vi "shag_start — 3.vi"() -> ()   [LabVIEW 2016]
uses:
  <vilib>/Instr/_visa.llb/VISA Configure Serial Port (Instr).vi
panel:
  in  "Блокировать зеркало №1":bool
  out "положение в мин 1":i32
  in  "stop":bool
  in  "all":T1(tab)
  out "положение шд":i32(knob) scale=-10.0..190.0
  out "текущее положение":string
  out "положение в минутах 1":string
  in  "Минуты":i32 min=-600 max=11400
  in  "Stop двигатель":bool
  in  "Вращение по градусам +":bool
  in  "Вращение по градусам -":bool
  in  "Вернуться в нулевое положение":bool
  in  "Задать текущее положение нулевым":bool
  in  "Установка минут":bool
  in  "Выберете COM порт":refnum<visa-resource-name>="COM1"
  in  "Скорость обмена данными":u32(ring)=19200 items=["9600"=9600, "19200"=19200, "38400"=38400, "57600"=57600]
  in  "Число бит на символ":u16=8 min=5 max=8 step=1
  in  "Контроль чётности":enum16{"None", "Odd", "Even", "Mark", "Space"}(ring)
  in  "Стоповый бит":u16(ring)=10 items=["1.0"=10, "1.5"=15, "2.0"=20]
  in  "Контроль переполнения":u16(ring) items=["None"=0, "XON/XOFF"=1, "RTS/CTS"=2, "DTR/DSR"=4]
  # "1 - адресс 1 двигателя\n2 - адресс 2 двигателя\n$0MV\\01+   - запуск всех двигателей в положительном направлении \n$0MS\\00   - остановка всех двигателей\n$0MJ\\04+\\00\\00\\01   - 1 шаг всех двигателей\n$0SS\\01\\10   - скорость 10 для всех двигателей"
  # "Зеркало №1:"
  # "Положение:"
  # "Ренгеновская трубка №2:"
  # "Положение ренгеновской трубк:"
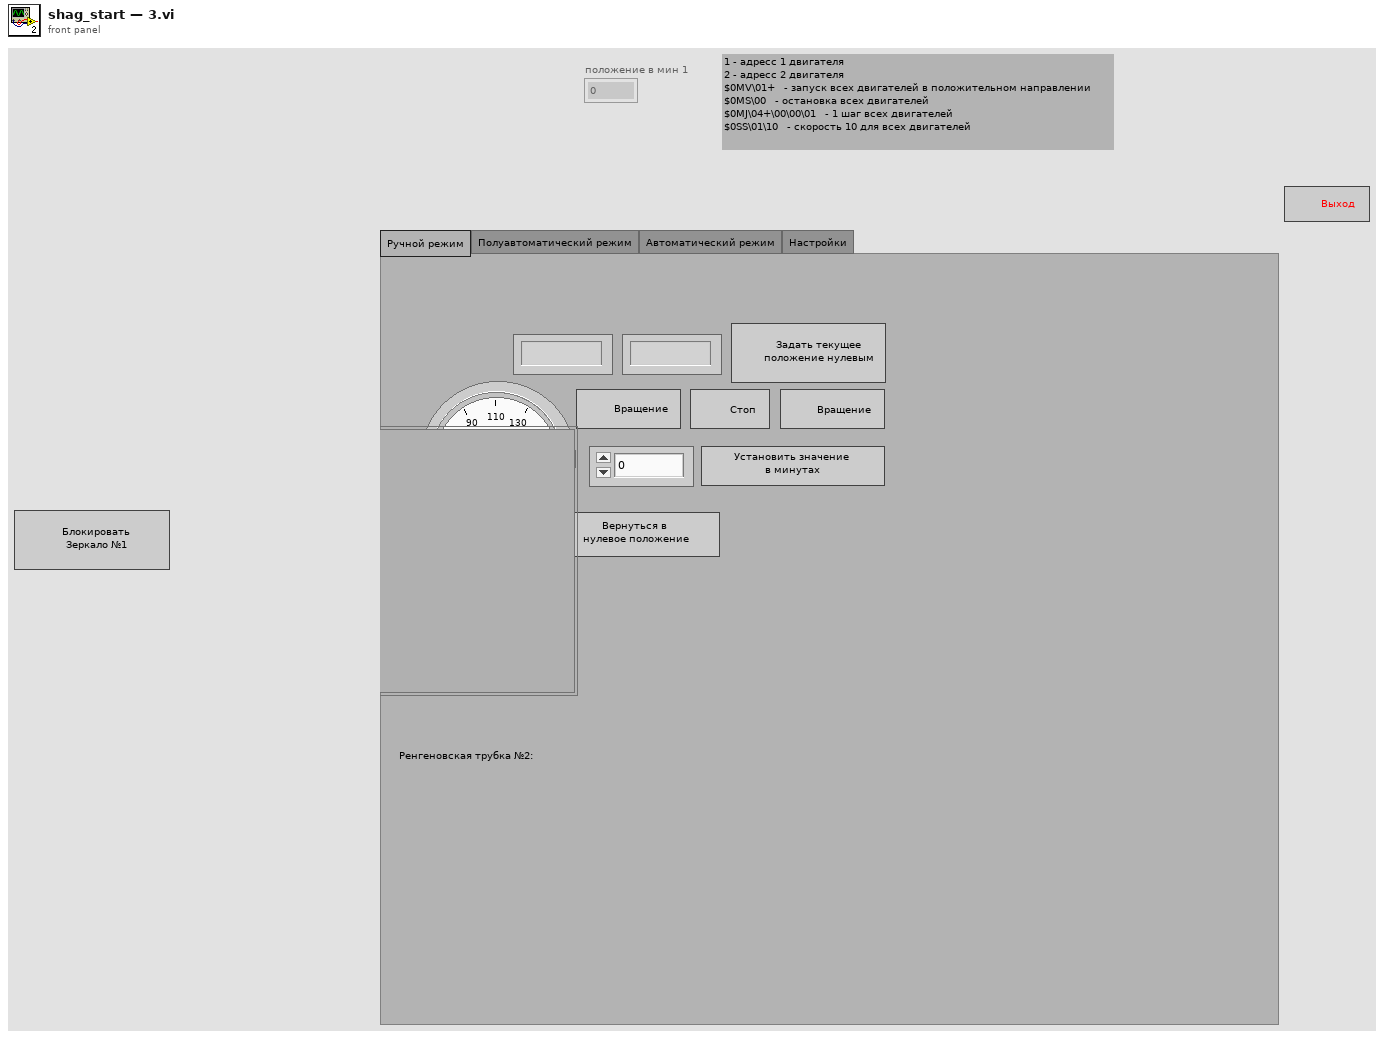
[diagram p1: front panel]
types:
  T1 = enum32{"Ручной режим", "Полуавтоматический режим", "Автоматический режим", "Настройки"}
  T2 = enum8{"Enabled", "Disabled", "Disabled and Grayed Out"}
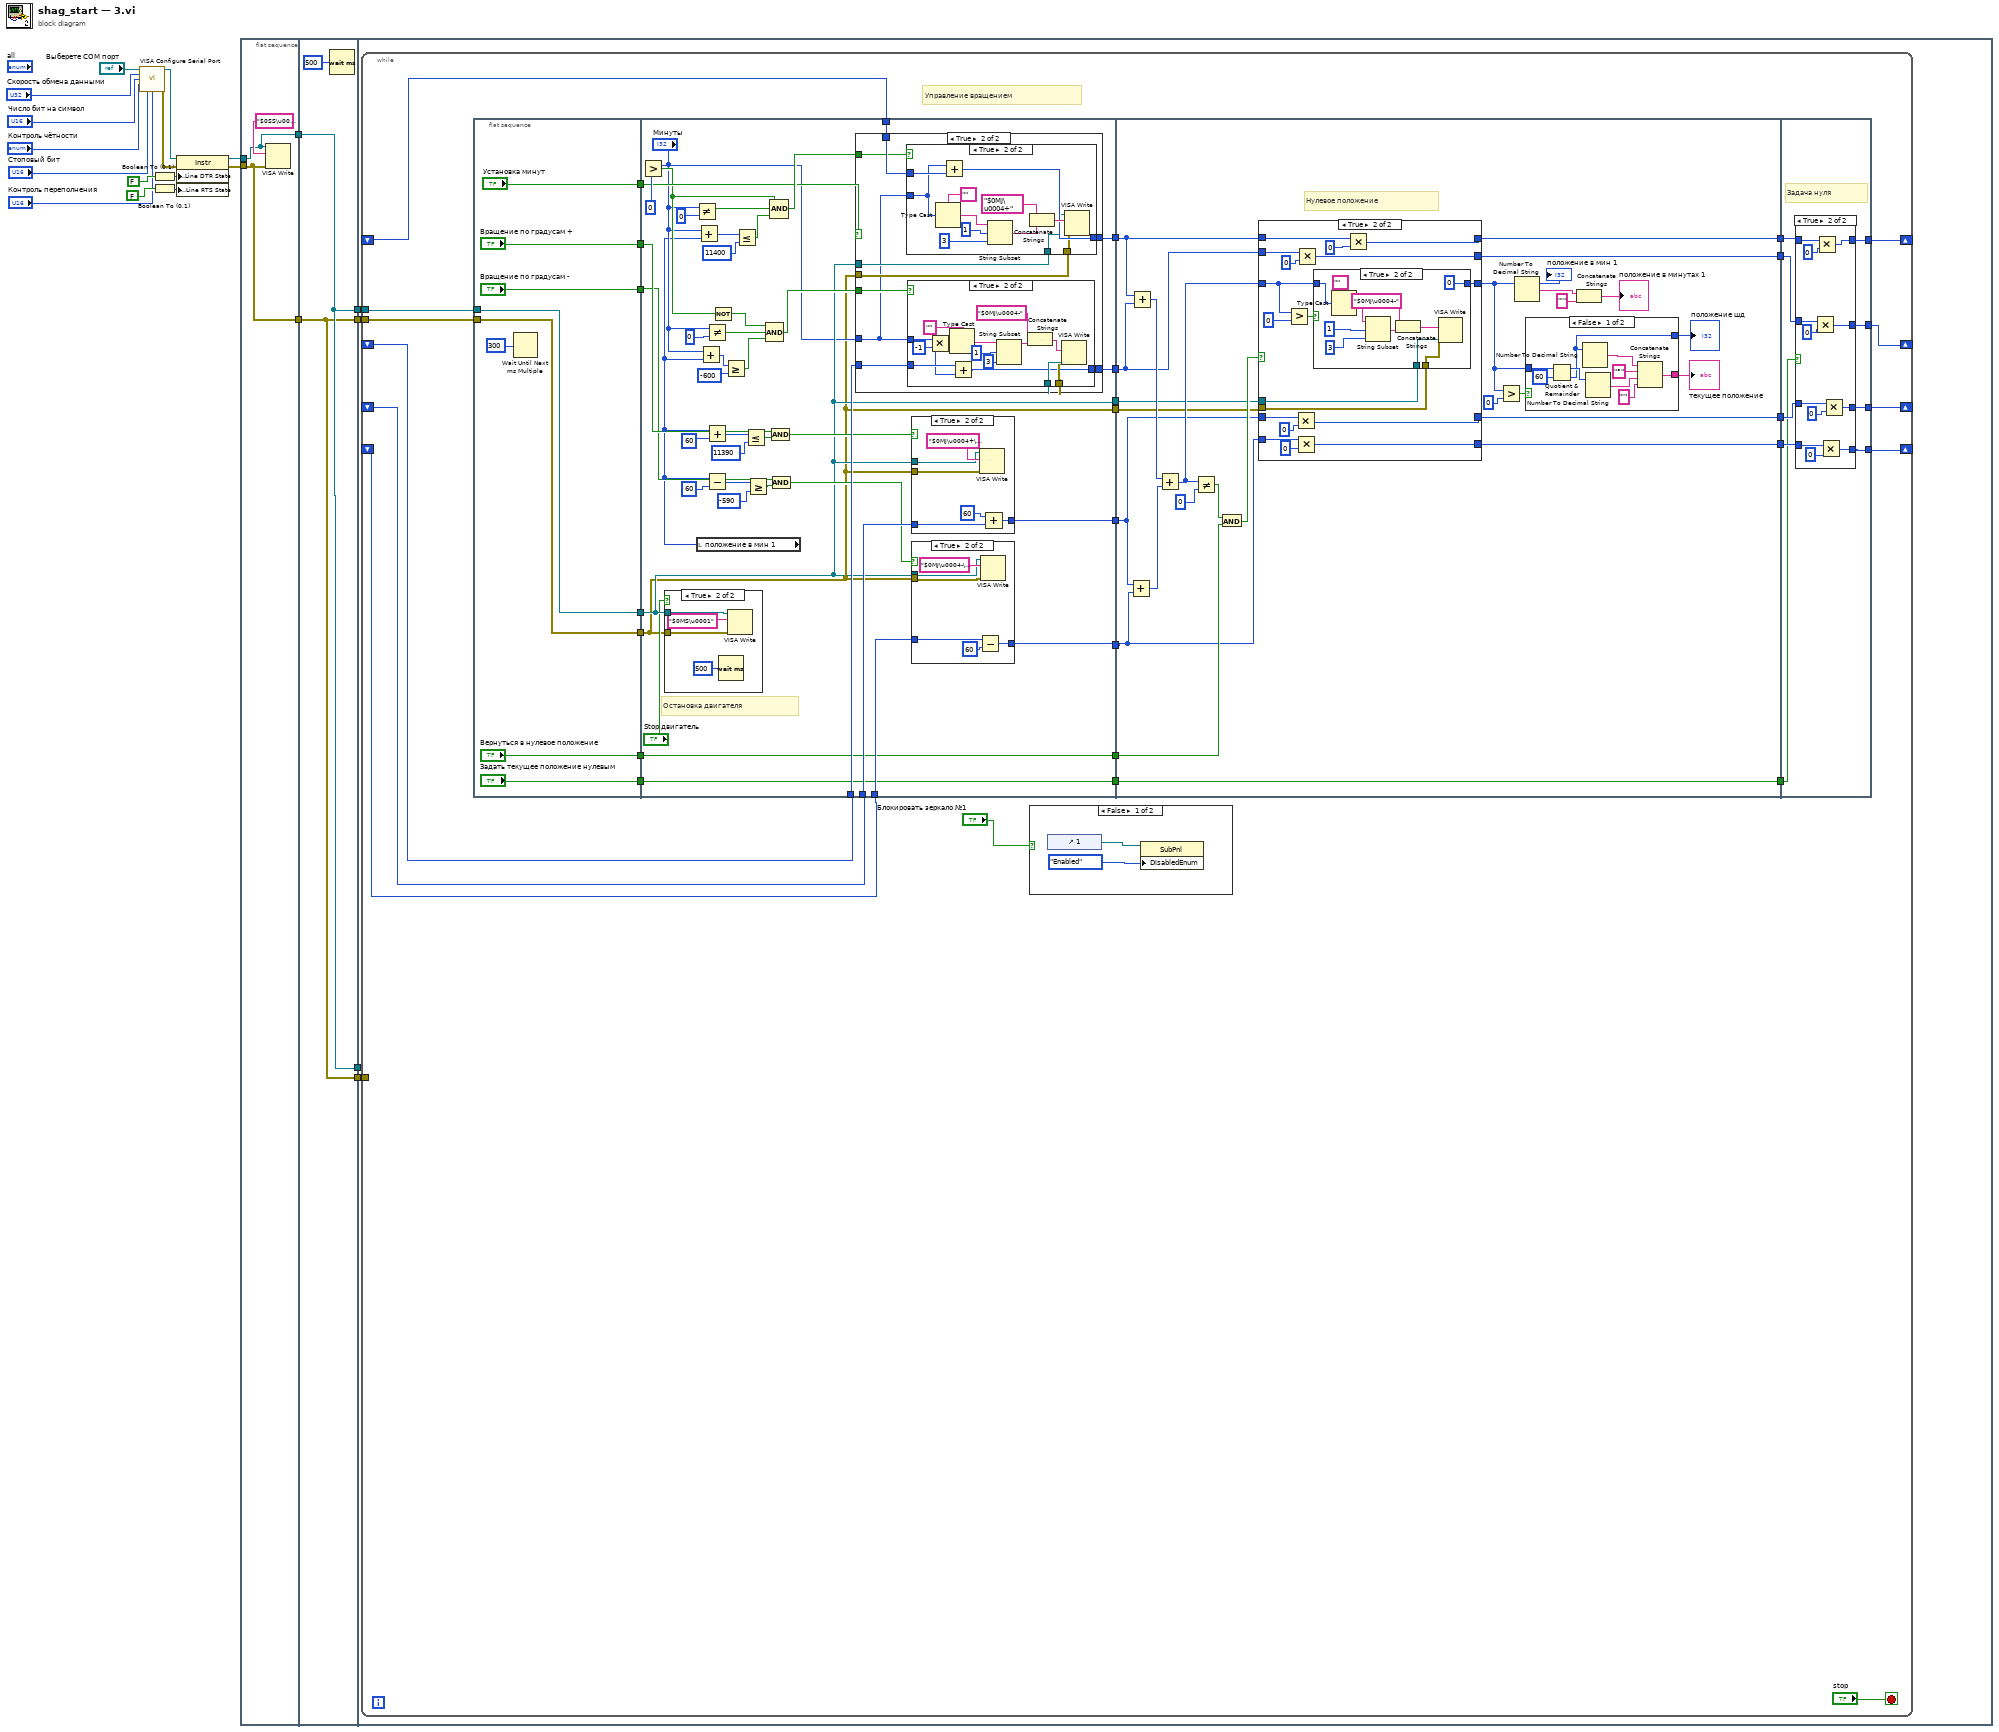
[diagram p0: block diagram]
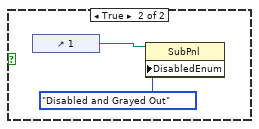
[diagram p2: hidden frame]
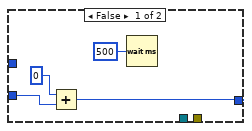
[diagram p4: hidden frame]
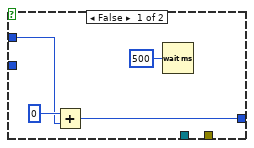
[diagram p5: hidden frame]
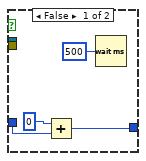
[diagram p7: hidden frame]
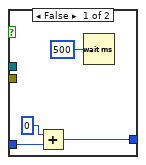
[diagram p8: hidden frame]
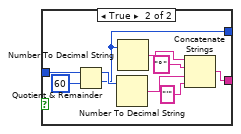
[diagram p9: hidden frame]
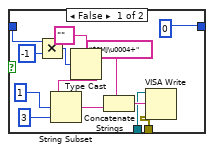
[diagram p11: hidden frame]
diagram:
  n1 = call-poly "VISA Configure Serial Port"("VISA resource name"="Выберете COM порт", "baud rate (9600)"="Скорость обмена данными", "data bits (8)"="Число бит на символ", "parity (0:none)"="Контроль чётности", "stop bits (10: 1 bit)"="Стоповый бит", "flow control (0:none)"="Контроль переполнения") -> ("VISA resource name out"=w18:refnum<visa-resource-name>, "error out"=w17:errorcluster)  [unwired: 8 in]
  n2 = Boolean To (0,1)(Boolean=FALSE ("DTR Write")) -> (0, 1=w19:i16)
  n3 = Boolean To (0,1)(Boolean=FALSE ("DTR Write")) -> (0, 1=w20:i16)
  n4 = property class="Instr"(reference=w18, error in=w17, "Serial Settings:Modem Line Settings:Line DTR State"=w19, "Serial Settings:Modem Line Settings:Line RTS State"=w20) -> (reference out=w16:refnum<visa-resource-name>, error out=w15:errorcluster)
  n5 = flat-sequence {
    tunnel: w16 -> [w22]
    tunnel: w15 -> [w21]
    tunnel: [w22] -> w13
    tunnel: [w21] -> w12
    tunnel: [w25] -> w14
    tunnel: w13 -> [w25]
    tunnel: w12 -> [w24]
    tunnel: [w24] -> w11
    tunnel: [w25] -> w2
    tunnel: [w24] -> w1
    tunnel: w14 -> [w29]
    tunnel: w11 -> [w28]
    tunnel: w2 -> [_]
    tunnel: w1 -> [w27]
    frame #0 {
      n6 = VISA Write(VISA resource name=w22, write buffer="$0SS\u0001\u0010", error in (no error)=w21) -> ()  [unwired: 3 out]
    }
    frame #1 {
      n7 = Wait (ms)(milliseconds to wait=u32 500) -> ()  [unwired: 1 out]
    }
    frame #2 {
      n8 = while {
        tunnel: w29 -> [w36]
        tunnel: w28 -> [w35]
        shift-right: [w31] -> _
        shift-left: _ -> [w40]
        shift-right: [w32] -> _
        shift-left: _ -> [w39]
        shift-right: [w33] -> _
        shift-left: _ -> [w38]
        shift-right: [w34] -> _
        shift-left: _ -> [w37]
        tunnel: w27 -> [_]
        stop <- "stop" stop-if-true
        # "Управление вращением"
        n9 = flat-sequence {
          tunnel: w35 -> [w72]
          tunnel: w36 -> [w73]
          tunnel: [w73] -> w60
          tunnel: [w72] -> w59
          tunnel: ["Вращение по градусам +"] -> w58
          tunnel: ["Вращение по градусам -"] -> w57
          tunnel: ["Вернуться в нулевое положение"] -> w56
          tunnel: ["Задать текущее положение нулевым"] -> w55
          tunnel: ["Установка минут"] -> w54
          tunnel: w60 -> [w93]
          tunnel: w59 -> [w74]
          tunnel: [w116] -> w53
          tunnel: w40 -> [w113]
          tunnel: w39 -> [w115]
          tunnel: [w114] -> w52
          tunnel: w38 -> [w112]
          tunnel: w37 -> [w111]
          tunnel: w58 -> [w97]
          tunnel: w57 -> [w96]
          tunnel: [w110] -> w51
          tunnel: [w109] -> w50
          tunnel: [w94] -> w49
          tunnel: w56 -> [w94]
          tunnel: [w74] -> w48
          tunnel: [w93] -> w47
          tunnel: [w92] -> w46
          tunnel: w55 -> [w92]
          tunnel: w54 -> [w86]
          tunnel: w53 -> [w190]
          tunnel: w52 -> [w191]
          tunnel: [w211] -> w45
          tunnel: [w209] -> w44
          tunnel: w51 -> [w192]
          tunnel: w50 -> [w193]
          tunnel: [w199] -> w43
          tunnel: [w207] -> w42
          tunnel: w49 -> [w203]
          tunnel: w48 -> [w198]
          tunnel: w47 -> [w197]
          tunnel: w46 -> [w195]
          tunnel: [w195] -> w41
          tunnel: [w285] -> w31
          tunnel: [w282] -> w32
          tunnel: w45 -> [w284]
          tunnel: w44 -> [w283]
          tunnel: [w281] -> w33
          tunnel: [w280] -> w34
          tunnel: w43 -> [w279]
          tunnel: w42 -> [w278]
          tunnel: w41 -> [w277]
          frame #0 {
            n10 = Wait Until Next ms Multiple(millisecond multiple=u32 300) -> ()  [unwired: 1 out]
          }
          frame #1 {
            # "Остановка двигателя"
            n11 = Greater?(x="Минуты", y=0) -> (0:w84:bool)
            n12 = case shown="True" "Stop двигатель" {
              tunnel: w93 -> [_ w163]
              tunnel: w74 -> [_ w162]
              frame False {
              }
              frame True {
                n13 = Wait (ms)(milliseconds to wait=u32 500) -> ()  [unwired: 1 out]
                n14 = VISA Write(VISA resource name=w163, write buffer="$0MS\u0001", error in (no error)=w162) -> ()  [unwired: 3 out]
              }
            }
            n15 = Not Equal?(x="Минуты", y=0) -> (x != y?=w83:bool)
            n16 = local read "положение в мин 1"() -> (w79:i32)
            n17 = Add(x="Минуты", y=w79) -> (x+y=w107:i32)
            n18 = Add(x="Минуты", y=w79) -> (x+y=w77:i32)
            n19 = Not Equal?(x="Минуты", y=0) -> (x != y?=w81:bool)
            n20 = Add(x=w79, y=60) -> (x+y=w102:i32)
            n21 = Subtract(x=w79, y=60) -> (x-y=w89:i32)
            n22 = Not(x=w84) -> (.not. x?=w85:bool)
            n23 = Greater Or Equal?(x=w77, y=-600) -> (x >= y?=w78:bool)
            n24 = Less Or Equal?(x=w107, y=11400) -> (x <= y?=w82:bool)
            n25 = Less Or Equal?(x=w102, y=11390) -> (x <= y?=w99:bool)
            n26 = Greater Or Equal?(x=w89, y=-590) -> (x >= y?=w90:bool)
            n27 = Compound Arithmetic op=AND(w85, w81, w78) -> (w103:bool)
            n28 = And(x=w97, y=w99) -> (x .and. y?=w98:bool)
            n29 = And(x=w96, y=w90) -> (x .and. y?=w95:bool)
            n30 = Compound Arithmetic op=AND(w84, w83, w82) -> (w105:bool)
            n31 = case shown="True" w86 {
              tunnel: [w118 w127] -> w116
              tunnel: w115 -> [w117 w126]
              tunnel: [w117 w125] -> w114
              tunnel: w113 -> [w118 w124]
              tunnel: w105 -> [_ w123]
              tunnel: w103 -> [_ w122]
              tunnel: w74 -> [_ w121]
              tunnel: w93 -> [_ w120]
              tunnel: "Минуты" -> [_ w119]
              frame False {
              }
              frame True {
                n32 = case shown="True" w123 {
                  tunnel: [w148 w154] -> w127
                  tunnel: w124 -> [w147 w153]
                  tunnel: w121 -> [_ w152]
                  tunnel: w120 -> [_ w151]
                  tunnel: w119 -> [_ w150]
                  frame False {
                    n33 = Add(x=0, y=w147) -> (x+y=w148:i32)
                    n34 = Wait (ms)(milliseconds to wait=u32 500) -> ()  [unwired: 1 out]
                  }
                  frame True {
                    n35 = Type Cast(type="", x=w150) -> (*(type *) &x=w157:string)
                    n36 = Add(x=w150, y=w153) -> (x+y=w154:i32)
                    n37 = String Subset(string=w157, offset (0)=1, length (rest)=3 ("length (rest)")) -> (substring=w156:string)
                    n38 = Concatenate Strings("$0MJ\u0004+" ("write buffer"), w156) -> (w160:string)
                    n39 = VISA Write(VISA resource name=w151, write buffer=w160, error in (no error)=w152) -> ()  [unwired: 3 out]
                  }
                }
                n40 = case shown="True" w122 {
                  tunnel: [w130 w136] -> w125
                  tunnel: w126 -> [w129 w135]
                  tunnel: w120 -> [_ w138]
                  tunnel: w121 -> [_ w137]
                  tunnel: w119 -> [_ w132]
                  frame False {
                    n41 = Add(x=0, y=w129) -> (x+y=w130:i32)
                    n42 = Wait (ms)(milliseconds to wait=u32 500) -> ()  [unwired: 1 out]
                  }
                  frame True {
                    n43 = Multiply(x=w132, y=-1) -> (x*y=w134:i32)
                    n44 = Type Cast(type="", x=w134) -> (*(type *) &x=w141:string)
                    n45 = Add(x=w135, y=w132) -> (x+y=w136:i32)
                    n46 = String Subset(string=w141, offset (0)=1, length (rest)=3 ("length (rest)")) -> (substring=w140:string)
                    n47 = Concatenate Strings("$0MJ\u0004-" ("write buffer"), w140) -> (w144:string)
                    n48 = VISA Write(VISA resource name=w138, write buffer=w144, error in (no error)=w137) -> ()  [unwired: 3 out]
                  }
                }
              }
            }
            n49 = case shown="True" w98 {
              tunnel: [w178 w185] -> w110
              tunnel: w112 -> [w177 w180]
              tunnel: w93 -> [_ w181]
              tunnel: w74 -> [_ w182]
              frame False {
                n50 = Add(x=0, y=w177) -> (x+y=w178:i32)
                n51 = Wait (ms)(milliseconds to wait=u32 500) -> ()  [unwired: 1 out]
              }
              frame True {
                n52 = VISA Write(VISA resource name=w181, write buffer="$0MJ\u0004+\u0000\u0000<", error in (no error)=w182) -> ()  [unwired: 3 out]
                n53 = Add(x=60, y=w180) -> (x+y=w185:i32)
              }
            }
            n54 = case shown="True" w95 {
              tunnel: [w168 w171] -> w109
              tunnel: w111 -> [w167 w170]
              tunnel: w93 -> [_ w174]
              tunnel: w74 -> [_ w173]
              frame False {
                n55 = Add(x=0, y=w167) -> (x+y=w168:i32)
                n56 = Wait (ms)(milliseconds to wait=u32 500) -> ()  [unwired: 1 out]
              }
              frame True {
                n57 = Subtract(x=w170, y=60 ("x")) -> (x-y=w171:i32)
                n58 = VISA Write(VISA resource name=w174, write buffer="$0MJ\u0004-\u0000\u0000<", error in (no error)=w173) -> ()  [unwired: 3 out]
              }
            }
          }
          frame #2 {
            # "Нулевое положение"
            n59 = Add(x=w192, y=w193) -> (x+y=w204:i32)
            n60 = Add(x=w190, y=w191) -> (x+y=w208:i32)
            n61 = Add(x=w208, y=w204) -> (x+y=w201:i32)
            n62 = Not Equal?(x=w201, y=0 ("x")) -> (x != y?=w200:bool)
            n63 = And(x=w200, y=w203) -> (x .and. y?=w210:bool)
            n64 = case shown="True" w210 {
              tunnel: [w232 w252] -> w189
              tunnel: w190 -> [w234 w249]
              tunnel: [w234 w248] -> w211
              tunnel: [w233 w247] -> w209
              tunnel: w201 -> [w232 w241]
              tunnel: [w230 w243] -> w207
              tunnel: [w231 w240] -> w199
              tunnel: w191 -> [w233 w239]
              tunnel: w198 -> [_ w238]
              tunnel: w197 -> [_ w237]
              tunnel: w192 -> [w231 w236]
              tunnel: w193 -> [w230 w235]
              frame False {
              }
              frame True {
                n65 = Greater?(x=w241, y=0) -> (0:w242:bool)
                n66 = Multiply(x=w236, y=0) -> (x*y=w240:i32)
                n67 = Multiply(x=w235, y=0) -> (x*y=w243:i32)
                n68 = Multiply(x=w239, y=0) -> (x*y=w247:i32)
                n69 = case shown="True" w242 {
                  tunnel: w241 -> [w257 w270]
                  tunnel: [0 0] -> w252
                  tunnel: w237 -> [w254 w267]
                  tunnel: w238 -> [w253 w266]
                  frame False {
                    n70 = Multiply(x=w257, y=-1) -> (x*y=w255:i32)
                    n71 = Type Cast(type="", x=w255) -> (*(type *) &x=w261:string)
                    n72 = String Subset(string=w261, offset (0)=1, length (rest)=3 ("length (rest)")) -> (substring=w260:string)
                    n73 = Concatenate Strings("$0MJ\u0004+" ("write buffer"), w260) -> (w264:string)
                    n74 = VISA Write(VISA resource name=w254, write buffer=w264, error in (no error)=w253) -> ()  [unwired: 3 out]
                  }
                  frame True {
                    n75 = Type Cast(type="", x=w270) -> (*(type *) &x=w273:string)
                    n76 = String Subset(string=w273, offset (0)=1, length (rest)=3 ("length (rest)")) -> (substring=w272:string)
                    n77 = Concatenate Strings("$0MJ\u0004-" ("write buffer"), w272) -> (w268:string)
                    n78 = VISA Write(VISA resource name=w267, write buffer=w268, error in (no error)=w266) -> ()  [unwired: 3 out]
                  }
                }
                n79 = Multiply(x=w249, y=0) -> (x*y=w248:i32)
              }
            }
            "положение в мин 1" <- w189
            n80 = Greater?(x=w189, y=0) -> (0:w206:bool)
            n81 = Number To Decimal String(number=w189) -> (decimal integer string=w187:string)  [unwired: 1 in]
            n82 = case shown="False" w206 {
              tunnel: w189 -> [w219 w229]
              tunnel: [w216 w223] -> w196
              tunnel: [w212 w221] -> w194
              frame False {
                n83 = Quotient & Remainder(x=w219, y=60) -> (x-y*floor(x/y)=w215:i32, floor(x/y)=w212:i32)
                n84 = Number To Decimal String(number=w212) -> (decimal integer string=w213:string)  [unwired: 1 in]
                n85 = Number To Decimal String(number=w215) -> (decimal integer string=w214:string)  [unwired: 1 in]
                n86 = Concatenate Strings(w213, "°" ("string"), w214, "'" ("string")) -> (w216:string)
              }
              frame True {
                n87 = Quotient & Remainder(x=w229, y=60) -> (x-y*floor(x/y)=w222:i32, floor(x/y)=w221:i32)
                n88 = Number To Decimal String(number=w222) -> (decimal integer string=w224:string)  [unwired: 1 in]
                n89 = Number To Decimal String(number=w221) -> (decimal integer string=w225:string)  [unwired: 1 in]
                n90 = Concatenate Strings(w225, "°" ("string"), w224, "'" ("string")) -> (w223:string)
              }
            }
            "положение шд" <- w194
            "текущее положение" <- w196
            n91 = Concatenate Strings(w187, "'" ("string")) -> (→"положение в минутах 1":string)
          }
          frame #3 {
            # "Задача нуля"
            n92 = case shown="True" w277 {
              tunnel: [w289 w300] -> w285
              tunnel: w284 -> [w289 w301]
              tunnel: w283 -> [w288 w297]
              tunnel: [w288 w296] -> w282
              tunnel: [w287 w293] -> w281
              tunnel: [w286 w292] -> w280
              tunnel: w279 -> [w287 w291]
              tunnel: w278 -> [w286 w290]
              frame False {
              }
              frame True {
                n93 = Multiply(x=w297, y=0) -> (x*y=w296:i32)
                n94 = Multiply(x=w301, y=0) -> (x*y=w300:i32)
                n95 = Multiply(x=w290, y=0) -> (x*y=w292:i32)
                n96 = Multiply(x=w291, y=0) -> (x*y=w293:i32)
              }
            }
          }
        }
        n97 = case shown="False" "Блокировать зеркало №1" {
          frame False {
            n98 = control-ref of="1"() -> (w62:refnum<vi>)
            n99 = property class="SubPnl"(reference=w62, "DisabledEnum"=T2."Enabled" ("Disabled")) -> ()  [unwired: 1 in, 2 out]
          }
          frame True {
            n100 = control-ref of="1"() -> (w64:refnum<vi>)
            n101 = property class="SubPnl"(reference=w64, "DisabledEnum"=T2."Disabled and Grayed Out" ("Disabled")) -> ()  [unwired: 1 in, 2 out]
          }
        }
      }
    }
  }
